vi "Read_coeff.vi"(5 "DevDet":i32=1, 6 "address":u32) -> (0 "A\n(Ax^2+Bx+C)":dbl, 1 "bck: a\n(ax+b)":dbl=465.88005, 2 "B\n(Ax^2+Bx+C)":dbl, 3 "C\n(Ax^2+Bx+C)":dbl, 4 "bck: b\n(ax+b)":dbl=465.88005)   [LabVIEW 2022 SP3]
uses:
  adcDLL_0001.dll
panel:
  out "InArray":u8[](array[numeric])
  out "string":string
  out "initialized array":u8[](array[numeric])
  # "Read calibration coefficients"
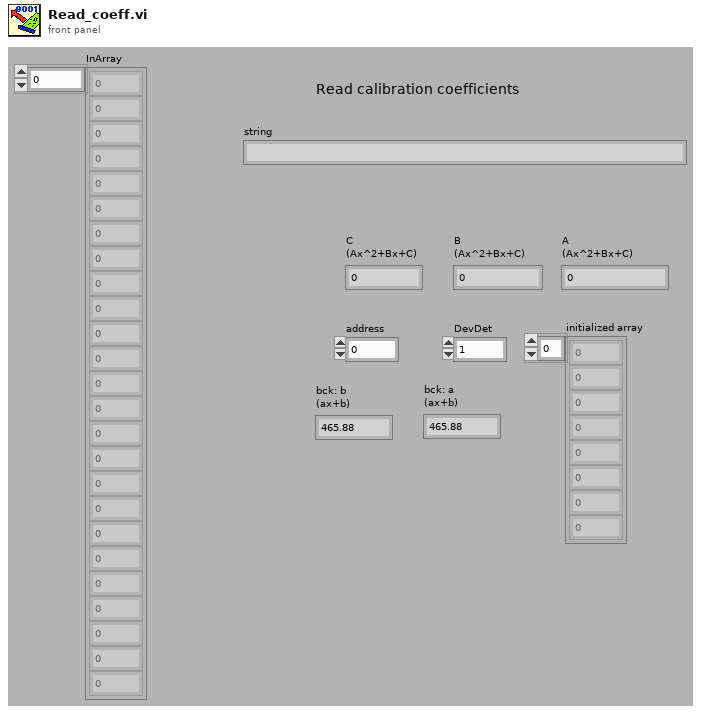
[diagram p1: front panel]
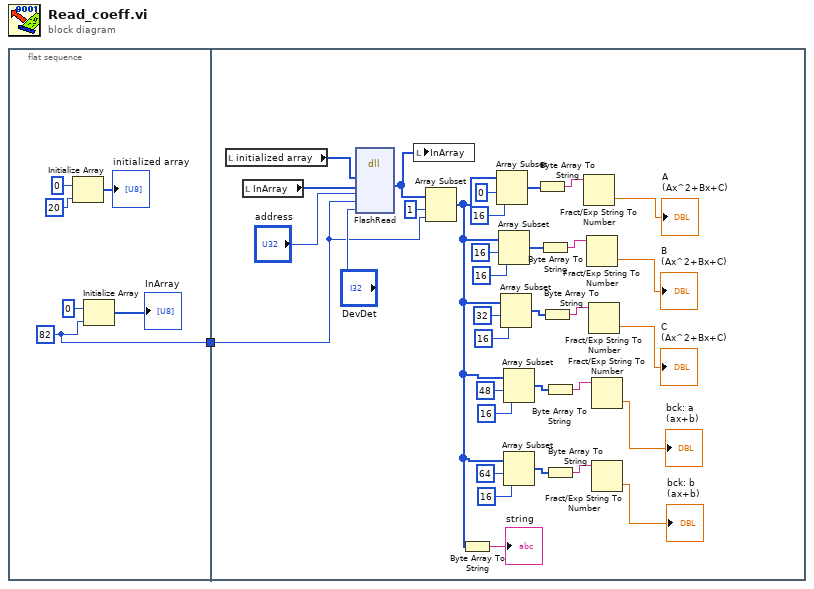
[diagram p0: block diagram]
diagram:
  n1 = flat-sequence {
    tunnel: [w2] -> w1
    tunnel: w1 -> [w36]
    frame #0 {
      w2 = 82 ("dimension size")
      n2 = Initialize Array(u8 0 ("element"), 20 ("dimension size")) -> (→"initialized array":u8[])
      n3 = Initialize Array(u8 0 ("element"), w2) -> (→"InArray":u8[])
    }
    frame #1 {
      n4 = local read "initialized array"() -> (w41:u8[])
      n5 = local read "InArray"() -> (w40:u8[])
      n6 = dll-call lib="D:/LabVIEWSuite_64_OS/Spectrometers/ASEQ LR1/adcDLL_0001.dll" fn="FlashRead"("OutputReport1"=w41, "InputData1"=w40, "address"="address", "length"=w36, "DevDet"="DevDet") -> ("InputData1"=w35:u8[])  [unwired: 8 in, 2 out]
      n7 = local write "InArray"(w35) -> ()
      n8 = Array Subset(array=w35, index=1, length=w36) -> (w8:u8[])
      n9 = Byte Array To String(unsigned byte array=w8) -> (string=→"string":string)
      n10 = Array Subset(array=w8, index=0, length=16) -> (w28:u8[])
      n11 = Array Subset(array=w8, index=16, length=16) -> (w24:u8[])
      n12 = Array Subset(array=w8, index=32, length=16) -> (w21:u8[])
      n13 = Array Subset(array=w8, index=48, length=16) -> (w15:u8[])
      n14 = Array Subset(array=w8, index=64, length=16) -> (w10:u8[])
      n15 = Byte Array To String(unsigned byte array=w28) -> (string=w27:string)
      n16 = Byte Array To String(unsigned byte array=w24) -> (string=w25:string)
      n17 = Byte Array To String(unsigned byte array=w21) -> (string=w22:string)
      n18 = Byte Array To String(unsigned byte array=w15) -> (string=w16:string)
      n19 = Byte Array To String(unsigned byte array=w10) -> (string=w11:string)
      n20 = Fract/Exp String To Number(string=w27) -> (number=→"A\n(Ax^2+Bx+C)":dbl)  [unwired: 3 in, 1 out]
      n21 = Fract/Exp String To Number(string=w25) -> (number=→"B\n(Ax^2+Bx+C)":dbl)  [unwired: 3 in, 1 out]
      n22 = Fract/Exp String To Number(string=w22) -> (number=→"C\n(Ax^2+Bx+C)":dbl)  [unwired: 3 in, 1 out]
      n23 = Fract/Exp String To Number(string=w16) -> (number=→"bck: a\n(ax+b)":dbl)  [unwired: 3 in, 1 out]
      n24 = Fract/Exp String To Number(string=w11) -> (number=→"bck: b\n(ax+b)":dbl)  [unwired: 3 in, 1 out]
    }
  }
